vi "COMI Get Dev Info.vi"(10 "pDevInfo":T1, 11 "hDevice":u32) -> (1 "function return":i32, 2 "pDevInfo out":T1, 3 "hDevice out":u32)   [LabVIEW 2017, in "Comidll.lvlib"]
doc: "int (COMI_GetDevInfo) (HANDLE hDevice, TComiDevInfo *pDevInfo);"
uses:
  <userlib>/Comidll/Comidll.lvlib
  <userlib>/Comidll/Comidll.dll
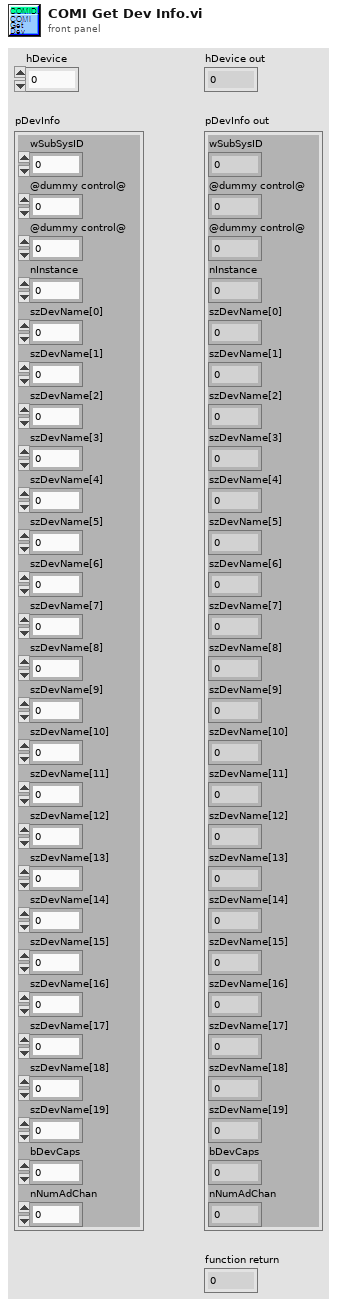
[diagram p1: front panel]
types:
  T1 = cluster{"wSubSysID":u16, "@dummy control@":i8, "@dummy control@":i8, "nInstance":u32, "szDevName[0]":i8, "szDevName[1]":i8, "szDevName[2]":i8, "szDevName[3]":i8, "szDevName[4]":i8, "szDevName[5]":i8, "szDevName[6]":i8, "szDevName[7]":i8, "szDevName[8]":i8, "szDevName[9]":i8, "szDevName[10]":i8, "szDevName[11]":i8, "szDevName[12]":i8, "szDevName[13]":i8, "szDevName[14]":i8, "szDevName[15]":i8, "szDevName[16]":i8, "szDevName[17]":i8, "szDevName[18]":i8, "szDevName[19]":i8, "bDevCaps":u8, "nNumAdChan":u8}
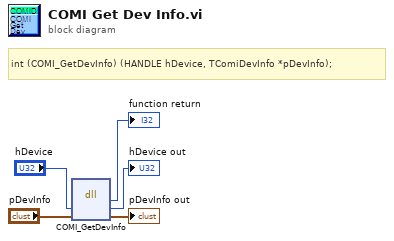
[diagram p0: block diagram]
diagram:
  # "int\t(COMI_GetDevInfo) (HANDLE hDevice, TComiDevInfo *pDevInfo);"
  n1 = dll-call lib="C:/Program Files/National Instruments/LabVIEW 2017/user.lib/Comidll/Comidll.*" fn="COMI_GetDevInfo"("hDevice"="hDevice", "pDevInfo"="pDevInfo") -> (→"function return":i32, "hDevice"=→"hDevice out":u32, "pDevInfo"=→"pDevInfo out":T1)  [unwired: 3 in, 2 out]
